vi "Test Base Clear Before Init Does Not Throw Error.vi"(8 "error in (no error)":errorcluster, 11 "Base Class Test In":refnum<class "Base Test.lvclass">) -> (0 "error out":errorcluster, 3 "Base Class Test Out":refnum<class "Base Test.lvclass">)   [LabVIEW 2020, in "Base Test.lvclass"]
uses:
  Base Test.lvclass
  C:/Program Files (x86)/National Instruments/LabVIEW 2020/vi.lib/Astemes/LUnit/Test Case.lvclass
  Base Test.lvclass/Base Test.ctl
  <vilib>/Astemes/LUnit/Test Case.lvclass/Test Case.ctl
  <vilib>/Astemes/LUnit/LUnit Assertion Result.lvclass/LUnit Assertion Result.ctl
  <vilib>/Astemes/LUnit/LUnit Test Case Result.lvclass/LUnit Test Case Result.ctl
  <vilib>/Astemes/LUnit/LUnit Method Result.lvclass/LUnit Method Result.ctl
  <vilib>/Astemes/LUnit/Palette/Pass.vi
  <vilib>/Astemes/LUnit/Palette/Fail.vi
  <vilib>/Astemes/LUnit/Set Assertion Type.vi
  <vilib>/Astemes/LUnit/Add test result.vi
  <vilib>/Astemes/LUnit/LUnit Write Passed.vi
  <vilib>/Astemes/LUnit/LUnit Write Message.vi
  <vilib>/Astemes/LUnit/LUnit Write Description.vi
  <vilib>/Astemes/LUnit/LUnit Write Assertion Type.vi
  <vilib>/Astemes/LUnit/LUnit Record Assertion Result.vi
  <vilib>/Astemes/LUnit/LUnit Aggregate Assertion Results.vi
  <vilib>/Astemes/LUnit/Assertion Result/LUnit Read Status.vi
  <vilib>/Astemes/LUnit/LUnit Read Message.vi
  <vilib>/Astemes/LUnit/LUnit Read Description.vi
  <vilib>/Astemes/LUnit/Method Result/LUnit Merge Status.vi
  <vilib>/Astemes/LUnit/LUnit Concatenate result strings.vi
  Framework/Base/Base.lvclass
  <vilib>/Astemes/LUnit/LUnit Assertion Result.lvclass
  <vilib>/Astemes/LUnit/Test Case.lvclass
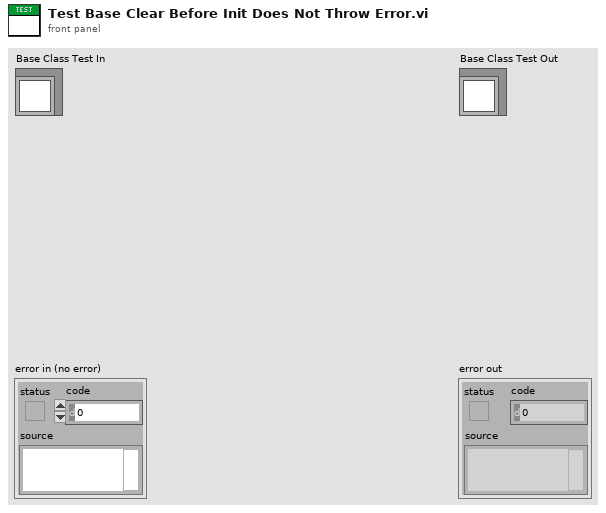
[diagram p1: front panel]
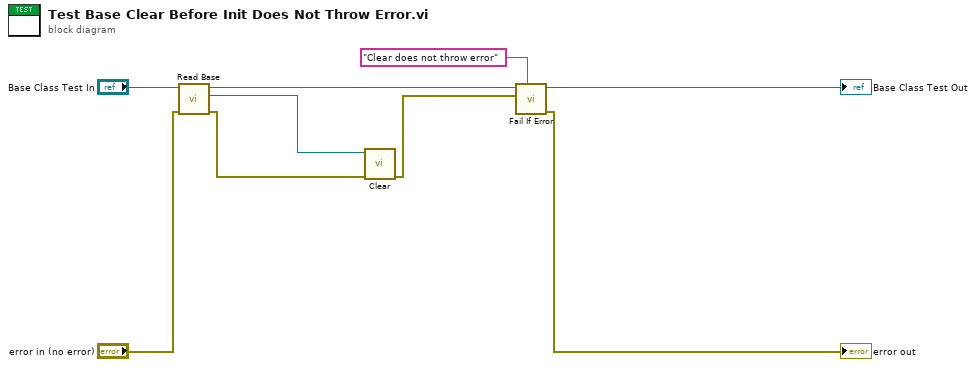
[diagram p0: block diagram]
diagram:
  n1 = call "Read Base.vi"("error in (no error)"="error in (no error)", "Base Class Test In"="Base Class Test In") -> ("error out"=w6:errorcluster, "Base.lvclass"=w7:refnum<class "Base.lvclass">, "Base Class Test Out"=w8:refnum<class "Base Test.lvclass">)  [unwired: 7 in]
  n2 = call-dynamic "Clear.vi"("error in (no error)"=w6, "Base In"=w7) -> ("error out"=w4:errorcluster)  [unwired: 9 in]
  n3 = call <vilib>:"Fail If Error.vi"("Description"="Clear does not throw error", "Assert error"=w4, "LUnit Test Case In"=w8) -> ("error out"=→"error out":errorcluster, "LUnit Test Case Out"=→"Base Class Test Out":refnum<class "Base Test.lvclass">)  [unwired: 7 in]
